vi "Add Project Items.vi"(8 "error in (no error)":errorcluster, 10 "Folder Location Ref":refnum<vi>, 11 "Module in":refnum<class "Module.lvclass">) -> (0 "error out":errorcluster, 3 "Module out":refnum<class "Module.lvclass">)   [LabVIEW 2025, in "Module.lvclass"]
doc: "Add items for the module required by the signal IP to the project."
uses:
  Module.lvclass
  Module.lvclass/Module.ctl
  Signal/Signal/Signal.lvclass
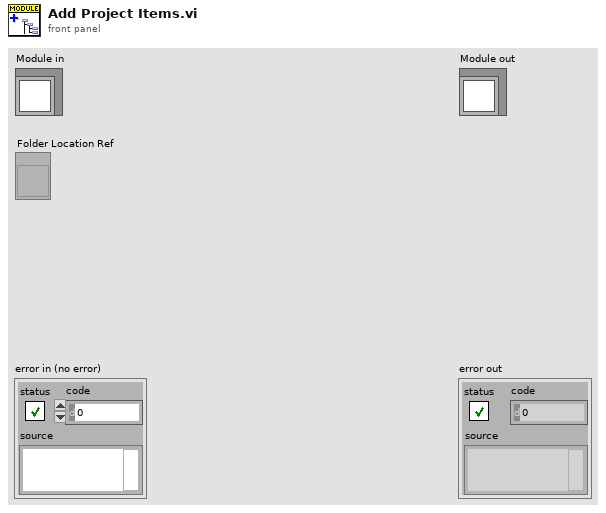
[diagram p1: front panel]
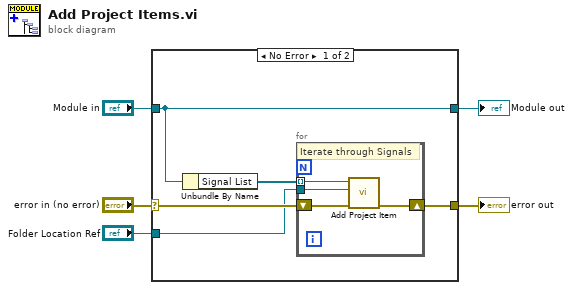
[diagram p0: block diagram]
diagram:
  n1 = case shown="No Error" "error in (no error)" {
    selector: "error in (no error)" -> [w8 w16]
    tunnel: [w7 w16] -> w4
    tunnel: [w10 w15] -> w2
    tunnel: "Module in" -> [w10 w15]
    tunnel: "Folder Location Ref" -> [w6 _]
    frame No Error {
      n2 = Unbundle By Name(w10) -> ("Signal List"=w9:refnum<class "Signal.lvclass">[])
      n3 = for {
        tunnel: w9 -> [w14] mode=indexing
        shift-right: [w12] -> w7
        shift-left: w8 -> [w13]
        tunnel: w6 -> [w11]
        # "Iterate through Signals"
        n4 = call-dynamic "Add Project Item.vi"("error in (no error)"=w13, "Folder Location Ref"=w11, "IO Class in"=w14) -> ("error out"=w12:errorcluster)  [unwired: 7 in, 1 out]
      }
    }
    frame Error {
    }
  }
  "error out" <- w4
  "Module out" <- w2
